vi "Configure Control Parameters.vi"(0 "VISA resource name":refnum<visa-resource-name>, 1 "Gain(P) (10.000)":dbl=10.0 min=0.001 max=1000.0 step=0.001 format="%.6f", 2 "Reset(I) (20)":dbl=20.0 min=0.0 max=10000.0 step=1.0 format="%.6f", 3 "Rate(D) (0)":dbl min=0.0 max=2500.0 step=1.0 format="%.6f", 5 "Output (0: sample heater)":u16(ring) items=["sample heater", "output 1 (warm-up heater) ", "output 2 (analog/still)"], 7 "Manual Output (0.000%)":dbl min=-100.0 max=100.0 step=0.001 format="%.3f", 9 "Heater Range (0: Off)":u16(ring) items=["Off", "31.6 uA", "100 uA", "316 uA", "1.00 mA", "3.16 mA", "10.0 mA", "31.6 mA", "100 mA"], 11 "error in (no error)":errorcluster) -> (4 "VISA resource name out":refnum<visa-resource-name>, 15 "error out":errorcluster)   [LabVIEW 2015, in "Lake Shore 372.lvlib"]
doc: "Configures the 372 Control Parameters. The VI uses <B>PID</B>, <B>MOUT</B>, and <B>RANGE</B>. PID sets the closed loop command parameters. MOUT sets the manual output heater percentage in current or power. The RANGE sets the current range for the heater.\n\nNotes:\nThe PID setting resolution is less than 6 digits indicated.\nThe range setting has no effect if an output is in the off mode, and does not apply to an output in monitor out mode. An output in monitor out mode is always on.\nPlease refer to Model 372 manual for further explanations."
uses:
  Lake Shore 372.lvlib
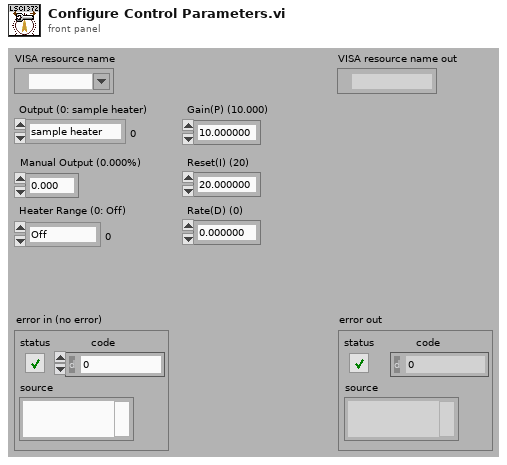
[diagram p1: front panel]
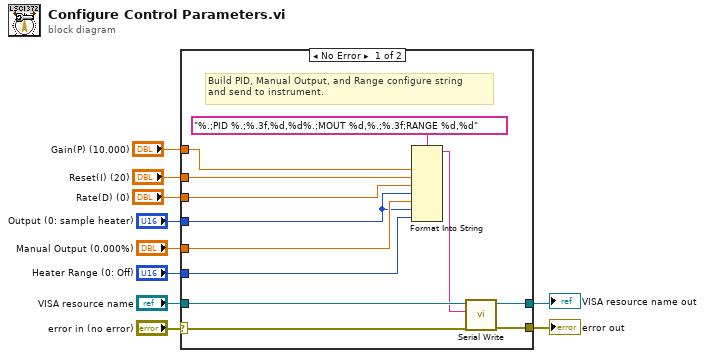
[diagram p0: block diagram]
diagram:
  n1 = case shown="No Error" "error in (no error)" {
    selector: "error in (no error)" -> [w14 w23]
    tunnel: "VISA resource name" -> [w22 w24]
    tunnel: [w21 w23] -> w9
    tunnel: [w20 w24] -> w8
    tunnel: "Manual Output (0.000%)" -> [w17 _]
    tunnel: "Heater Range (0: Off)" -> [w16 _]
    tunnel: "Output (0: sample heater)" -> [w15 _]
    tunnel: "Rate(D) (0)" -> [w11 _]
    tunnel: "Gain(P) (10.000)" -> [w13 _]
    tunnel: "Reset(I) (20)" -> [w12 _]
    frame No Error {
      # "Build PID, Manual Output, and Range configure string\nand send to instrument."
      n2 = Format Into String(format string="%.;PID %.;%.3f,%d,%d%.;MOUT %d,%.;%.3f;RANGE %d,%d", w13, w12, w11, w15, w17, w15, w16) -> (resulting string=w18:string)  [unwired: 2 in, 1 out]
      n3 = call "Serial Write.vi"("error in (no error)"=w14, "Write Buffer (\"\")"=w18, "VISA resource name"=w22) -> ("error out"=w21:errorcluster, "VISA resource name out"=w20:refnum<visa-resource-name>)  [unwired: 6 in, 1 out]
    }
    frame Error {
    }
  }
  "error out" <- w9
  "VISA resource name out" <- w8
